vi "RohdeSchwarz ZNB ReadSpectrum.vi"(5 "Continuar":bool=TRUE, 6 "Formato Traza":i32(ring) items=["dB Mag", "Phase", "Smith", "Polar", "Delay", "SWR", "Lin Mag", "Real", "Imag", "Inverted Smith", "Unwrapped Phase"], 7 "Fichero":path=path "C:/Users/pemar/Documents/LabVIEW Data/PruebaSAI.txt", 8 "error in (no error)":errorcluster, 10 "MeasConfig":T1={"Tiempo (sec)"=0.0, "Campo X (T)"=0.0, "Campo Y (T)"=10.0, "Campo Z (T)"=0.025, "Temperatura (K)"=300.0, "Start Frequency (Hz)"=1000000.0, "Stop Frequency (Hz)"=4000000000.0, "IF Bandwidth"=10000.0, "Sweep time(s)"=600.0, "Meas Points"=10000, "Power Level (0.0)"=-10.0} {"Campo Z (T)" format="%.2e"; "Campo Y (T)" format="%.2e"; "Sweep time(s)" format="%^.2g"; "Temperatura (K)" format="%.2e"; "Campo X (T)" format="%.2e"; "Tiempo (sec)" format="%^.2g"; "Start Frequency (Hz)" format="%.2e"; "Stop Frequency (Hz)" format="%.2e"; "IF Bandwidth" format="%.2e"; "Power Level (0.0)" format="%^.2g"}, 11 "visa VNA":refnum<visa-resource-name>="ZNB20-62-101710") -> (0 "error out":errorcluster, 1 "XY Graph":cluster{dbl[], dbl[]}(graph))   [LabVIEW 2017]
doc: "See readme.txt for more details."
uses:
  RohdeSchwarz ZNB MeasConfig.ctl
  <vilib>/Utility/file.llb/Write Delimited Spreadsheet (DBL).vi
  <instrlib>/Rohde&Schwarz Vector Network Analyzer/Rohde&Schwarz Vector Network Analyzer.lvlib
panel:
  out "Estado":string
  out "VISA resource name 2":refnum<visa-resource-name>="ZNB20-62-101710"
  out "measuredData":dbl[][](array[numeric])
  out "num points":i32
  in  "Display":bool=TRUE
  in  "ID Query":bool=TRUE
  in  "Reset Device":bool=TRUE
  # "Rohde & Schwarz Vector Network Analyzer: Single Sweep Mode"
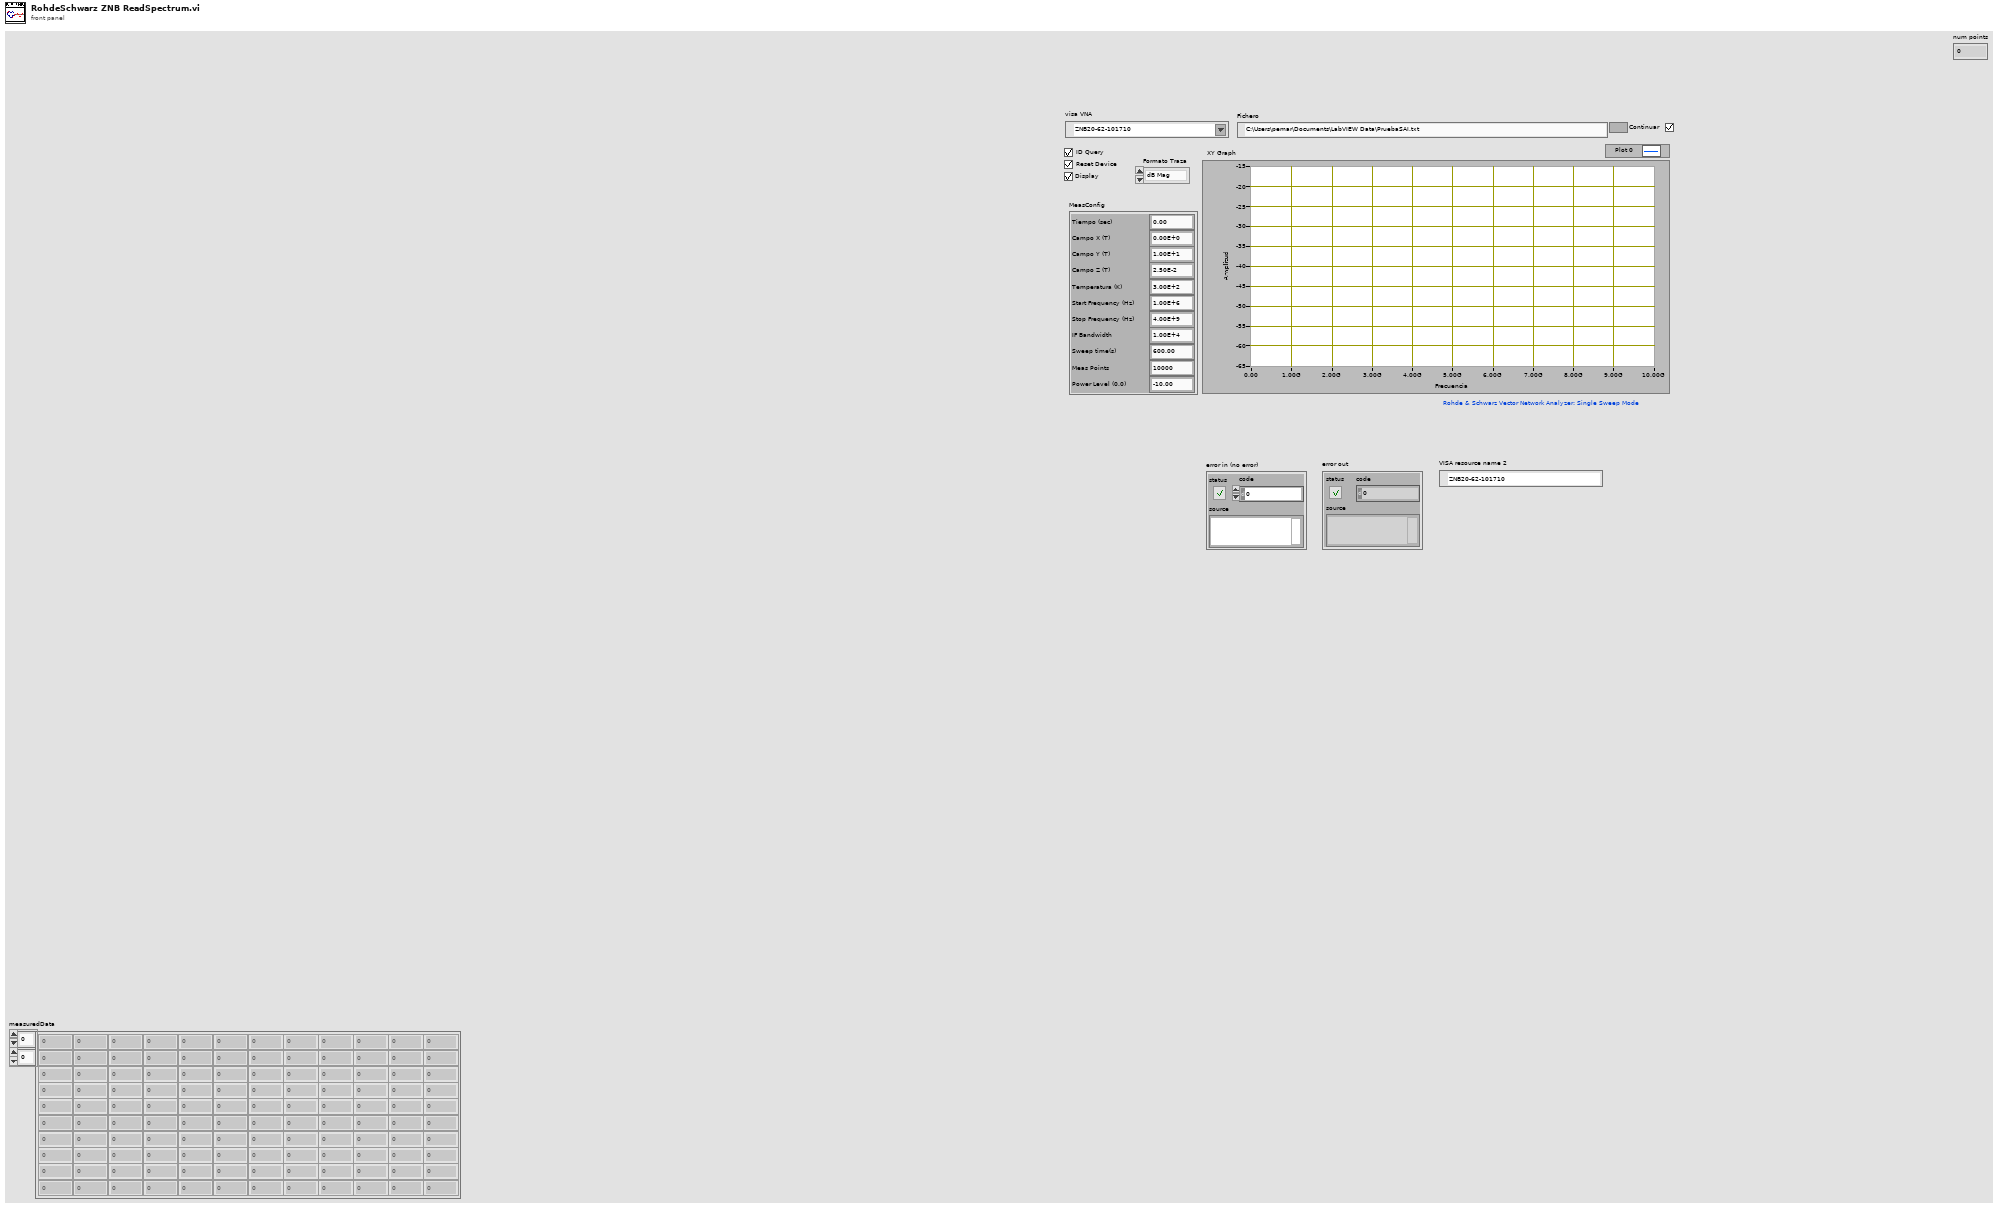
[diagram p1: front panel]
types:
  T1 = typedef "RohdeSchwarz ZNB MeasConfig.ctl" = cluster{"Tiempo (sec)":dbl, "Campo X (T)":dbl, "Campo Y (T)":dbl, "Campo Z (T)":dbl, "Temperatura (K)":dbl, "Start Frequency (Hz)":dbl, "Stop Frequency (Hz)":dbl, "IF Bandwidth":dbl, "Sweep time(s)":dbl, "Meas Points":i32, "Power Level (0.0)":dbl}
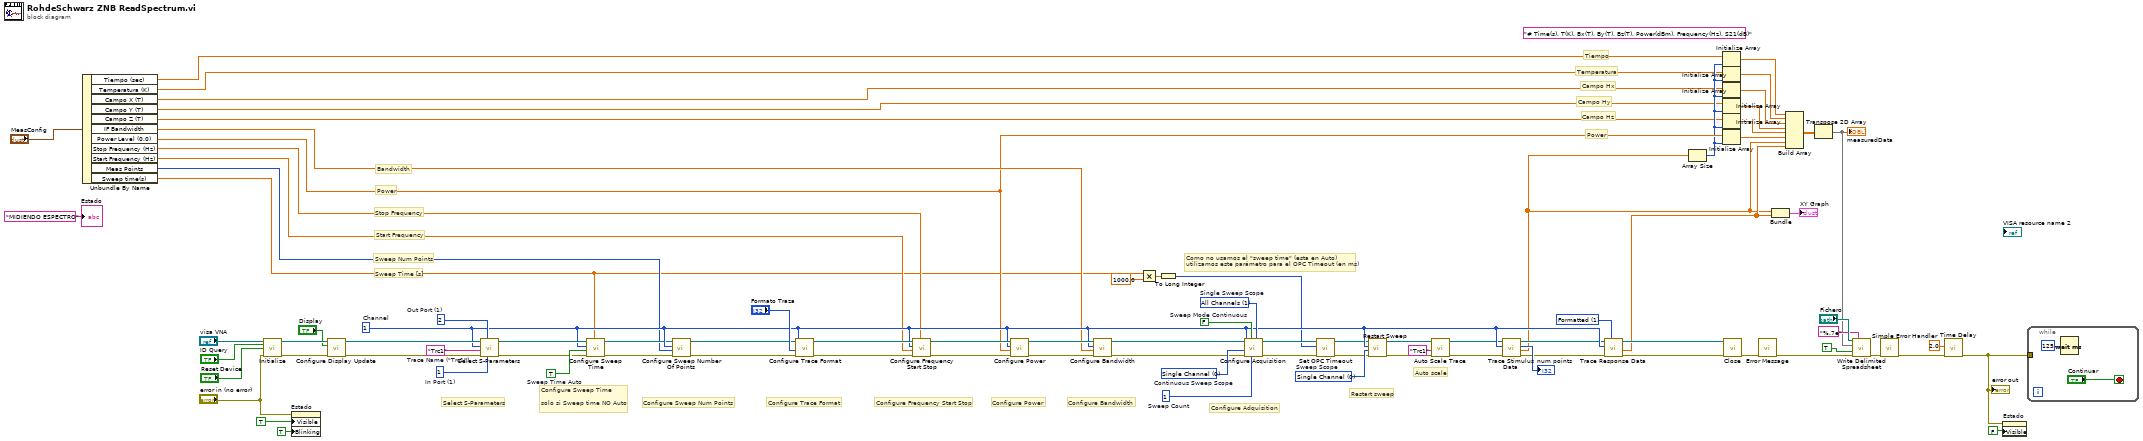
[diagram p0: block diagram]
diagram:
  (unwired) "# Time(s), T(K), Bx(T), By(T), Bz(T), Power(dBm), Frequency(Hz), S21(dB)" ("format string")
  w53 = 1 items=["Unformatted", "Formatted", "Unformatted With Trace Mathematics"] ("Data Format (Unformatted)")
  w77 = 1  # Sweep Count
  w61 = "Trc1"  # Trace Name ("Trc1")
  w62 = 1  # In Port (1)
  w63 = 2  # Out Port (1)
  w80 = 0 items=["Single Channel", "All Channels"]  # Sweep Scope
  w81 = TRUE  # Sweep Time Auto
  w58 = 1  # Channel
  w82 = 0 items=["Single Channel", "All Channels"]  # Continuous Sweep Scope
  w83 = FALSE  # Sweep Mode Continuous
  w84 = 1 items=["Single Channel", "All Channels"]  # Single Sweep Scope
  # "Campo Hy"
  # "Campo Hz"
  # "Como no usamos el \"sweep time\" (esta en Auto)\nutilizamos este parámetro para el OPC Timeout (en ms)"
  # "Sweep Time [s]"
  # "Sweep Num Points"
  # "Start Frequency"
  # "Stop Frequency"
  # "Power"
  # "Bandwidth"
  # "Tiempo"
  # "Temperatura"
  # "Campo Hx"
  # "Power"
  # "Auto scale"
  # "Restart sweep"
  # "Configure Adquisition"
  # "Configure Sweep Num Points"
  # "Configure Bandwidth"
  # "Select S-Parameters"
  # "Configure Power"
  # "Configure Sweep Time\n\nsolo si Sweep time NO Auto"
  # "Configure Trace Format"
  # "Configure Frequency Start Stop"
  n1 = Unbundle By Name("MeasConfig") -> ("Tiempo (sec)"=w5:dbl, "Temperatura (K)"=w4:dbl, "Campo X (T)"=w3:dbl, "Campo Y (T)"=w2:dbl, "Campo Z (T)"=w1:dbl, "IF Bandwidth"=w45:dbl, "Power Level (0.0)"=w41:dbl, "Stop Frequency (Hz)"=w44:dbl, "Start Frequency (Hz)"=w43:dbl, "Meas Points"=w42:i32, "Sweep time(s)"=w21:dbl)
  n2 = call <instrlib>:"Initialize.vi"("VISA resource name"="visa VNA", "ID Query (T: Check)"="ID Query", "Reset (T: Reset)"="Reset Device", "error in (no error)"="error in (no error)") -> ("VISA resource name out"=w89:refnum<visa-resource-name>, "error out"=w88:errorcluster)  [unwired: 10 in]
  n3 = property on="Estado" class="Str"(error in="error in (no error)", "Visible"=TRUE, "Blinking"=TRUE) -> ()  [unwired: 1 in, 2 out]
  n4 = call <instrlib>:"Configure Display Update.vi"("error in (no error)"=w88, "Display In Remote (F)"="Display", "VISA resource name"=w89) -> ("error out"=w67:errorcluster, "VISA resource name out"=w66:refnum<visa-resource-name>)  [unwired: 7 in]
  n5 = call <instrlib>:"Select S-Parameters.vi"("In Port (1)"=w62, "Out Port (1)"=w63, "error in (no error)"=w67, "Trace Name (\"Trc1\")"=w61, "Channel (1)"=w58, "VISA resource name"=w66) -> ("error out"=w64:errorcluster, "VISA resource name out"=w65:refnum<visa-resource-name>)  [unwired: 4 in]
  n6 = call <instrlib>:"Configure Sweep Time.vi"("Sweep Time (21.909e-3)"=w21, "error in (no error)"=w64, "Auto Sweep Time (T)"=w81, "Channel (1)"=w58, "VISA resource name"=w65) -> ("error out"=w60:errorcluster, "VISA resource name out"=w57:refnum<visa-resource-name>)  [unwired: 5 in]
  n7 = call <instrlib>:"Configure Sweep Number Of Points.vi"("error in (no error)"=w60, "Number Of Points (201)"=w42, "Channel (1)"=w58, "VISA resource name"=w57) -> ("error out"=w59:errorcluster, "VISA resource name out"=w56:refnum<visa-resource-name>)  [unwired: 6 in]
  n8 = call <instrlib>:"Configure Trace Format.vi"("error in (no error)"=w59, "Format (dB Mag)"="Formato Traza", "Channel (1)"=w58, "VISA resource name"=w56) -> ("error out"=w75:errorcluster, "VISA resource name out"=w74:refnum<visa-resource-name>)  [unwired: 6 in]
  n9 = call <instrlib>:"Configure Frequency Start Stop.vi"("Stop Frequency (4GHz)"=w44, "error in (no error)"=w75, "Start Frequency (300kHz)"=w43, "Channel (1)"=w58, "VISA resource name"=w74) -> ("error out"=w73:errorcluster, "VISA resource name out"=w72:refnum<visa-resource-name>)  [unwired: 5 in]
  n10 = call <instrlib>:"Configure Power.vi"("error in (no error)"=w73, "Power (-10.0)"=w41, "Channel (1)"=w58, "VISA resource name"=w72) -> ("error out"=w71:errorcluster, "VISA resource name out"=w70:refnum<visa-resource-name>)  [unwired: 6 in]
  n11 = call <instrlib>:"Configure Bandwidth.vi"("error in (no error)"=w71, "Bandwidth (10kHz)"=w45, "Channel (1)"=w58, "VISA resource name"=w70) -> ("error out"=w69:errorcluster, "VISA resource name out"=w68:refnum<visa-resource-name>)  [unwired: 6 in]
  n12 = Multiply(x=w21, y=1000.0) -> (x*y=w20:dbl)
  n13 = To Long Integer(number=w20) -> (32bit integer=w18:i32)
  n14 = call <instrlib>:"Configure Acquisition.vi"("Single Sweep Scope (All Channels)"=w84, "Sweep Count (1)"=w77, "Sweep Mode Continuous (F)"=w83, "error in (no error)"=w69, "Continuous Sweep Scope (All Channels)"=w82, "Channel (1)"=w58, "VISA resource name"=w68) -> ("error out"=w24:errorcluster, "VISA resource name out"=w25:refnum<visa-resource-name>)  [unwired: 3 in]
  n15 = call <instrlib>:"Set OPC Timeout.vi"("error in (no error)"=w24, "OPC Timeout"=w18, "VISA resource name"=w25) -> ("error out"=w23:errorcluster, "VISA resource name out"=w22:refnum<visa-resource-name>)  [unwired: 7 in]
  n16 = call <instrlib>:"Restart Sweep.vi"("error in (no error)"=w23, "Sweep Scope (All Channels)"=w80, "Channel (1)"=w58, "VISA resource name"=w22) -> ("error out"=w38:errorcluster, "VISA resource name out"=w37:refnum<visa-resource-name>)  [unwired: 6 in]
  n17 = call <instrlib>:"Auto Scale Trace.vi"("error in (no error)"=w38, "Trace Name (\"\")"="Trc1" ("Trace Name (\"\")"), "VISA resource name"=w37) -> ("error out"=w34:errorcluster, "VISA resource name out"=w33:refnum<visa-resource-name>)  [unwired: 7 in]
  n18 = call <instrlib>:"Trace Stimulus Data.vi"("error in (no error)"=w34, "Channel (1)"=w58, "VISA resource name"=w33) -> ("error out"=w35:errorcluster, "Trace Data"=w28:dbl[], "No of Values"=→"num points":i32, "VISA resource name out"=w32:refnum<visa-resource-name>)  [unwired: 5 in]
  n19 = call <instrlib>:"Trace Response Data.vi"("Data Format (Unformatted)"=w53, "error in (no error)"=w35, "Channel (1)"=w58, "VISA resource name"=w32) -> ("error out"=w30:errorcluster, "Trace Data"=w29:dbl[], "VISA resource name out"=w31:refnum<visa-resource-name>)  [unwired: 4 in, 1 out]
  n20 = Array Size(array=w28) -> (size(s)=w8:i32)
  n21 = Initialize Array(w5, w8) -> (w11:dbl[])
  n22 = Initialize Array(w4, w8) -> (w10:dbl[])
  n23 = Initialize Array(w3, w8) -> (w9:dbl[])
  n24 = Initialize Array(w2, w8) -> (w7:dbl[])
  n25 = Initialize Array(w1, w8) -> (w6:dbl[])
  n26 = Initialize Array(w41, w8) -> (w48:dbl[])
  n27 = call <instrlib>:"Close.vi"("error in (no error)"=w30, "VISA resource name"=w31) -> ("error out"=w76:errorcluster)  [unwired: 9 in]
  n28 = call <instrlib>:"Error Message.vi"("error in (no error)"=w76) -> ("error out"=w39:errorcluster)  [unwired: 10 in, 4 out]
  n29 = Bundle("Trace Data"=w28, "Trace Data"=w29) -> (→"XY Graph":cluster{"Trace Data":dbl[], "Trace Data":dbl[]})  [unwired: 1 in]
  n30 = Build Array(w11, w10, w9, w7, w6, w48, w28, w29) -> (w47:dbl[][])
  n31 = Transpose 2D Array(2D array=w47) -> (transposed array=w40:dbl[][])
  "measuredData" <- w40
  n32 = call-poly <vilib>:"Write Delimited Spreadsheet.vi"("file path (dialog if empty)"="Fichero", "format (%.3f)"="%.7e", "2D data"=w40, "append to file? (new file:F)"=TRUE, "error in (no error)"=w39) -> ("error out"=w51:errorcluster)  [unwired: 9 in, 1 out]
  n33 = call <vilib>:"Simple Error Handler.vi"("error in (no error)"=w51) -> ("error out"=w27:errorcluster)  [unwired: 4 in, 4 out]
  n34 = call "Time Delay"("error in (no error)"=w27, "Delay Time (s)"=2.0) -> ("error out"=w15:errorcluster)  [unwired: 9 in]
  "error out" <- w15
  n35 = property on="Estado" class="Str"(error in=w15, "Visible"=FALSE) -> ()  [unwired: 1 in, 2 out]
  n36 = while {
    tunnel: w15 -> [_]
    stop <- "Continuar" stop-if-true
    n37 = Wait (ms)(milliseconds to wait=u32 125) -> ()  [unwired: 1 out]
  }
  "Estado" <- "MIDIENDO ESPECTRO" ("Estado")
